vi "read TBM configuration.vi"(8 "error in":errorcluster, 11 "Logic Sequencer editor node in":refnum<class "Logic Sequencer editor node.lvclass">) -> (0 "error out":errorcluster, 2 "configuration":refnum<class "TBM configuration.lvclass">, 3 "Logic Sequencer editor node out":refnum<class "Logic Sequencer editor node.lvclass">)   [LabVIEW 2013, in "Logic Sequencer editor node.lvclass"]
uses:
  Logic Sequencer editor node.lvclass
  <vilib>/NI/Tag Bus Module Framework/root configuration/TBM configuration.lvclass
  Logic Sequencer editor node.lvclass/Logic Sequencer editor node.ctl
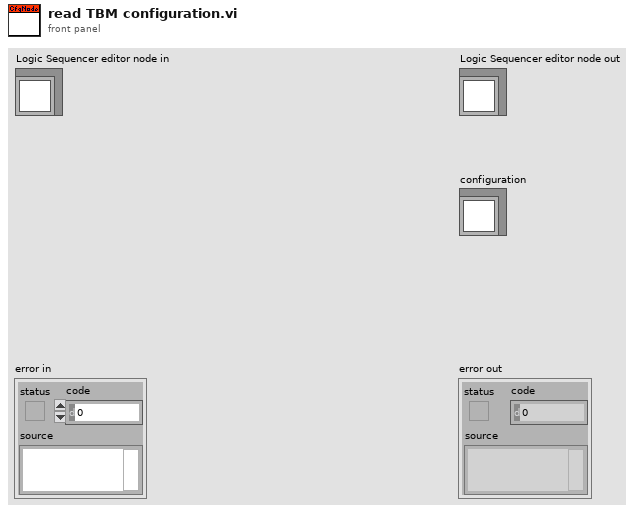
[diagram p1: front panel]
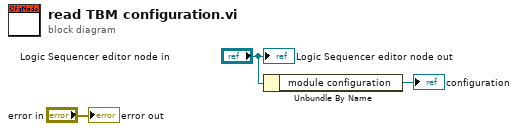
[diagram p0: block diagram]
diagram:
  n1 = Unbundle By Name("Logic Sequencer editor node in") -> ("module configuration"=→"configuration":refnum<class "Logic Sequencer configuration.lvclass">)
  "error out" <- "error in"
  "Logic Sequencer editor node out" <- "Logic Sequencer editor node in"
